vi "Shutdown Core.vi"(8 "error in (no error)":errorcluster, 11 "Test Consumer in":refnum<class "Test Consumer.lvclass">) -> (0 "error out":errorcluster, 3 "Test Consumer out":refnum<class "Test Consumer.lvclass">)   [LabVIEW 2017, in "Test Consumer.lvclass"]
uses:
  Test Consumer.lvclass
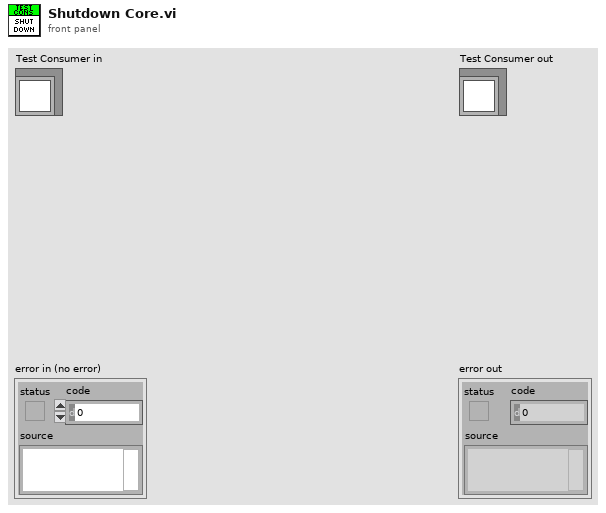
[diagram p1: front panel]
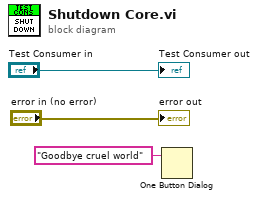
[diagram p0: block diagram]
diagram:
  n1 = One Button Dialog(message="Goodbye cruel world") -> ()  [unwired: 1 in, 1 out]
  "error out" <- "error in (no error)"
  "Test Consumer out" <- "Test Consumer in"
